vi "Plugin.Initialize Transceiver.vi"(7 "transceiver settings":T1, 8 "error in (no error)":errorcluster, 9 "Transfer Groups Configurations":refnum<class "Transfer Group Configuration.lvclass">[](array[class]), 10 "component classes":refnum<class>[](array[class]), 11 "Plugin in":refnum<class "Plugin.lvclass">) -> (0 "error out":errorcluster, 2 "Transceiver":refnum<class "Transceiver.lvclass">, 3 "Plugin out":refnum<class "Plugin.lvclass">)   [LabVIEW 2017, in "DSF Core.lvlib" / "Plugin.lvclass"]
uses:
  Plugin.lvclass
  Shared/Classes/Transfer Group/Transfer Group Configuration.lvclass
  Transceiver/Transceiver.lvclass
  DSF Configuration API/Public/Controls/DSF Settings Info.ctl
  DSF Core.lvlib
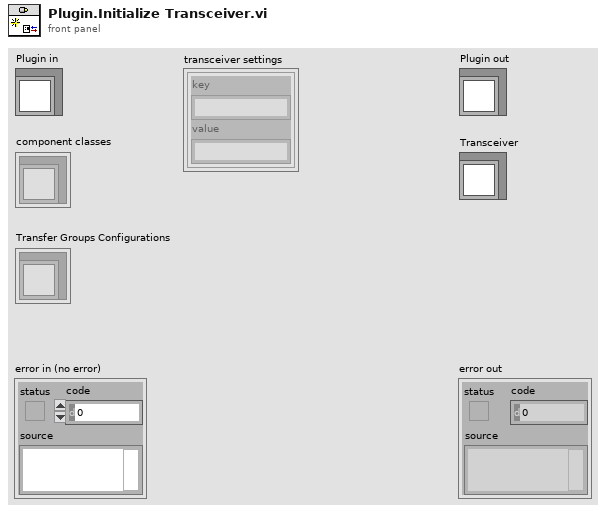
[diagram p1: front panel]
types:
  T1 = typedef "DSF Core.lvlib/DSF Settings Info.ctl" = cluster{"key":string, "value":string}[]
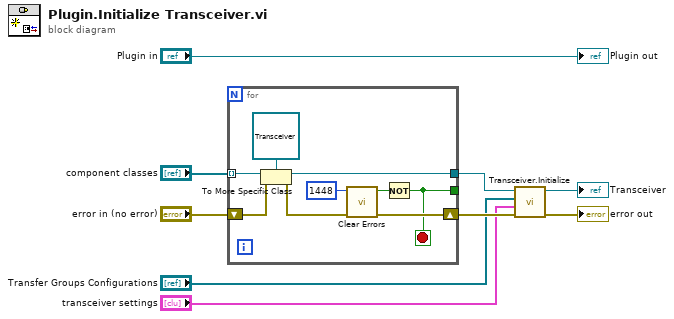
[diagram p0: block diagram]
diagram:
  n1 = for {
    tunnel: "component classes" -> [w17] mode=indexing
    tunnel: [w16] -> w5
    shift-right: [w13] -> w6
    shift-left: "error in (no error)" -> [w12]
    tunnel: [w10] -> _
    stop <- w10 stop-if-true
    n2 = To More Specific Class(target class=refnum<class "Transceiver.lvclass"> refnum ("DSF.Engine.lvlib:Transceiver"), reference=w17, error in=w12) -> (specific class reference=w16:refnum<class "Transceiver.lvclass">, error out=w14:errorcluster)
    n3 = call <vilib>:"Clear Errors.vi"("error in (no error)"=w14, "specific error code to clear (0: all)"=1448) -> ("error out"=w13:errorcluster, "specific error cleared?"=w11:bool)  [unwired: 4 in]
    n4 = Not(x=w11) -> (.not. x?=w10:bool)
  }
  n5 = call-dynamic "Transceiver.Initialize.vi"("error in (no error)"=w6, "transceiver settings"="transceiver settings", "Transfer Groups Configurations"="Transfer Groups Configurations", "Transceiver in"=w5) -> ("error out"=→"error out":errorcluster, "Transceiver out"=→"Transceiver":refnum<class "Transceiver.lvclass">)  [unwired: 6 in]
  "Plugin out" <- "Plugin in"
